vi "SysLog PC store messages.vi"(8 "Fehler (in)":errorcluster caption="Fehlerkonstante") -> (0 "Fehler (out)":errorcluster caption="Fehlerkonstante")   [LabVIEW 2015, in "SysLog.lvlib"]
doc: "Speichern der gesammelten Fehlermeldungen in die\n#ErrLogHistory Dateie - laut angegebenem Pfad.\nBaut ein TextArray mit Zwischenzeilen.\nriw 8.6.2018"
uses:
  SysLog.lvlib
  Aktionen FGV SysLog.ctl
  Allgemein/allgemeine Sub-VIs.lvlib
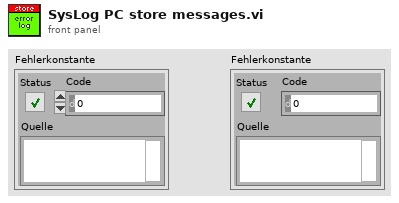
[diagram p1: front panel]
types:
  T1 = typedef "SysLog.lvlib/Aktionen FGV SysLog.ctl" = enum16{"initialisieren", "lesen", "schreiben", "history button ref"}
  T2 = enum16{"open", "replace", "create", "open or create", "replace or create", "replace or create with confirmation"}
  T3 = cluster{"Anzeige Array":bool[], "Message Array":string[], "SysLog Incon Array":enum16{"OK", "Warnung", "Fehler"}[], "Status Message Array":string[], "Status SysLog Incon Array":enum16{"OK", "Warnung", "Fehler"}[]}
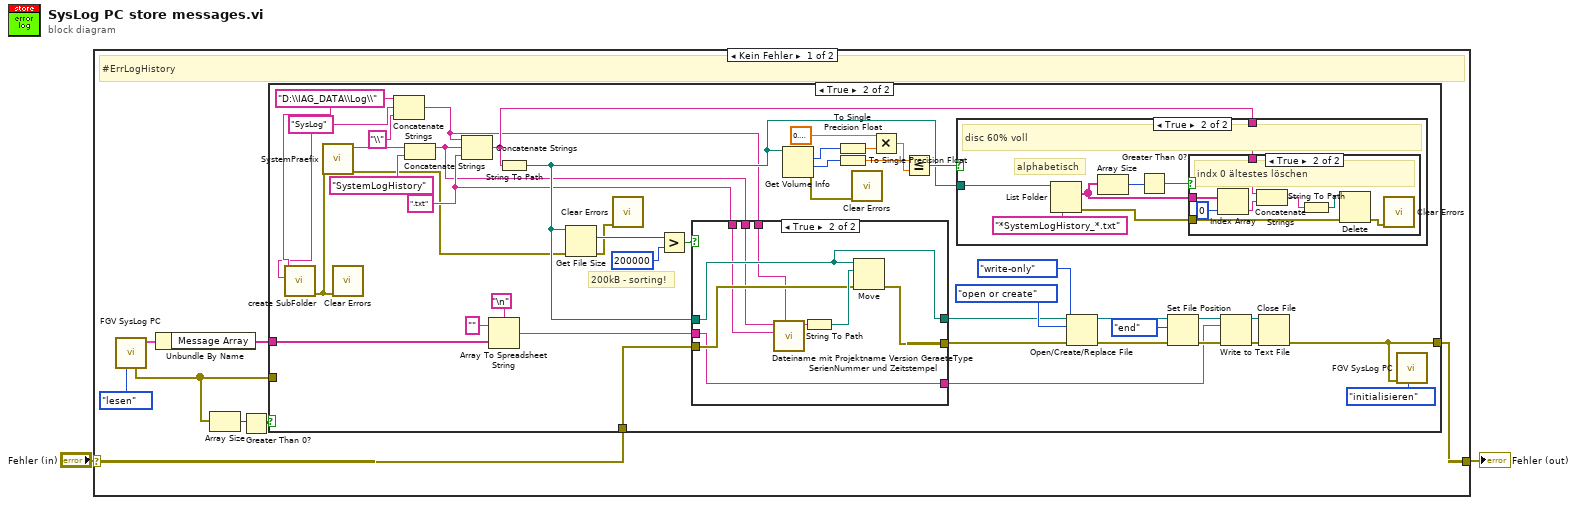
[diagram p0: block diagram]
diagram:
  n1 = case shown="Kein Fehler" "Fehler (in)" {
    selector: "Fehler (in)" -> [w9 w81]
    tunnel: [w8 w81] -> w1
    frame No Error {
      # "#ErrLogHistory"
      n2 = call "FGV SysLog PC.vi"("Aktion"=Aktionen_FGV_SysLog."lesen") -> ("Anzeige Cluster"=w5:T3, "Fehler out"=w4:errorcluster[])  [unwired: 7 in, 2 out]
      n3 = Unbundle By Name(w5) -> ("Message Array"=w3:string[])
      n4 = Array Size(array=w4) -> (size(s)=w7:i32)
      n5 = Greater Than 0?(x=w7) -> (x > 0?=w6:bool)
      n6 = case shown="True" w6 {
        tunnel: w4 -> [_ _]
        tunnel: w9 -> [_ w33]
        tunnel: [_ w32] -> w8
        tunnel: w3 -> [_ w17]
        frame False {
        }
        frame True {
          w14 = "SysLog"
          w15 = "D:\\IAG_DATA\\Log\\"
          w20 = ".txt" ("Dateiname")
          # "200kB - sorting!"
          n7 = call "create SubFolder.vi"("Ordner"=w14, "Pfad"=w15) -> ("Fehler (Ausgang)"=w13:errorcluster)  [unwired: 9 in]
          n8 = call "SystemPraefix.vi"("Fehler (Eingang)"=w13) -> ("Fehler (Ausgang)"=w12:errorcluster, "SystemPraefix"=w21:string)  [unwired: 9 in]
          n9 = call <vilib>:"Clear Errors.vi"("error in (no error)"=w13) -> ()  [unwired: 5 in, 2 out]
          n10 = Concatenate Strings(w15, w14, "\\" ("String")) -> (w16:string)
          n11 = Concatenate Strings(w21, "SystemLogHistory" ("Dateiname")) -> (w18:string)
          n12 = Concatenate Strings(w16, w18, w20) -> (w22:string)
          n13 = Array To Spreadsheet String(delimiter (Tab)="\n", array=w17, 3:"" ("Format-String")) -> (spreadsheet string=w34:string)
          n14 = String To Path(string=w22) -> (path=w23:path)
          n15 = Get File Size(file=w23, error in=w12) -> (size (in bytes)=w49:i64, 0:w48:errorcluster)  [unwired: 1 out]
          n16 = call <vilib>:"Clear Errors.vi"("error in (no error)"=w48) -> ()  [unwired: 5 in, 2 out]
          n17 = Greater?(x=w49, y=i64 200000) -> (0:w36:bool)
          n18 = case shown="True" w36 {
            tunnel: w34 -> [w70 w76]
            tunnel: w23 -> [w71 w77]
            tunnel: w33 -> [w69 w79]
            tunnel: w18 -> [_ w75]
            tunnel: w20 -> [_ w74]
            tunnel: [w69 w78] -> w38
            tunnel: [w71 w77] -> w35
            tunnel: [w70 w76] -> w37
            tunnel: w16 -> [_ w72]
            frame False {
            }
            frame True {
              n19 = call "Dateiname mit Projektname Version GeraeteType SerienNummer und Zeitstempel.vi"("Pfad"=w72, "Extension in"=w74, "File Name in"=w75) -> ("File Name"=w73:string)  [unwired: 8 in]
              n20 = String To Path(string=w73) -> (path=w80:path)
              n21 = Move(source path=w77, error in=w79, 10:w80) -> (error out=w78:errorcluster)  [unwired: 2 in, 2 out]
            }
          }
          n22 = Get Volume Info(11:w23) -> (0:w24:errorcluster, 1:w31:i64, 2:w30:i64)  [unwired: 1 in, 3 out]
          n23 = To Single Precision Float(number=w30) -> (single precision float=w26:sgl)
          n24 = To Single Precision Float(number=w31) -> (single precision float=w27:sgl)
          n25 = call <vilib>:"Clear Errors.vi"("error in (no error)"=w24) -> ()  [unwired: 5 in, 2 out]
          n26 = Multiply(x=sgl 0.4, y=w26) -> (x*y=w28:sgl)
          n27 = Less Or Equal?(x=w27, y=w28) -> (x <= y?=w25:bool)
          n28 = case shown="True" w25 {
            tunnel: w23 -> [_ w60]
            tunnel: w22 -> [_ w54]
            frame False {
            }
            frame True {
              # "alphabetisch"
              # "disc 60% voll"
              n29 = List Folder(path=w60, pattern="*SystemLogHistory_*.txt" ("Muster")) -> (filenames=w56:string[], error out=w59:errorcluster)  [unwired: 2 in, 2 out]
              n30 = Array Size(array=w56) -> (size(s)=w55:i32)
              n31 = Greater Than 0?(x=w55) -> (x > 0?=w57:bool)
              n32 = case shown="True" w57 {
                tunnel: w59 -> [_ w68]
                tunnel: w56 -> [_ w66]
                tunnel: w54 -> [_ w62]
                frame False {
                }
                frame True {
                  # "indx 0 ältestes löschen"
                  n33 = Index Array(array=w66, index=0 ("Index")) -> (element=w64:string)
                  n34 = Concatenate Strings(w62, w64) -> (w63:string)
                  n35 = String To Path(string=w63) -> (path=w65:path)
                  n36 = Delete(path (use dialog)=w65, error in=w68) -> (error out=w67:errorcluster)  [unwired: 3 in, 2 out]
                  n37 = call <vilib>:"Clear Errors.vi"("error in (no error)"=w67) -> ()  [unwired: 5 in, 2 out]
                }
              }
            }
          }
          n38 = Open/Create/Replace File(file path (use dialog)=w35, error in=w38, operation (0:open)=T2."open or create" ("Operation (0:Öffnen)"), access (0:read/write)=enum16{"read/write", "read-only", "write-only"}."write-only" ("Zugriff (0:Lesen/Schreiben)")) -> (refnum out=w42:refnum<file>, error out=w41:errorcluster)  [unwired: 2 in, 1 out]
          n39 = Set File Position(refnum=w42, from (0:start)=enum16{"start", "end", "current"}."end", error in=w41) -> (refnum out=w40:refnum<file>, error out=w39:errorcluster)  [unwired: 1 in]
          n40 = Write to Text File(file (use dialog)=w40, text=w37, error in=w39) -> (refnum out=w47:refnum<file>, error out=w46:errorcluster)  [unwired: 1 in, 1 out]
          n41 = Close File(refnum=w47, error in=w46) -> (error out=w32:errorcluster)  [unwired: 1 out]
          n42 = call "FGV SysLog PC.vi"("Aktion"=Aktionen_FGV_SysLog."initialisieren", "Fehler (in)"=w32) -> ()  [unwired: 6 in, 4 out]
        }
      }
    }
    frame Error {
    }
  }
  "Fehler (out)" <- w1
